vi "Write Focus.vi"(8 "error in (no error)":errorcluster, 10 "GSdevice.lvclass":refnum<class "GSdevice.lvclass">, 11 "GSserver in":refnum<class "GSserver.lvclass">) -> (0 "error out":errorcluster, 3 "GSserver out":refnum<class "GSserver.lvclass">)   [LabVIEW 2018, in "GSserver.lvclass"]
uses:
  GSserver.lvclass
  GSdevice/GSdevice.lvclass
  GSserver.lvclass/GSserver.ctl
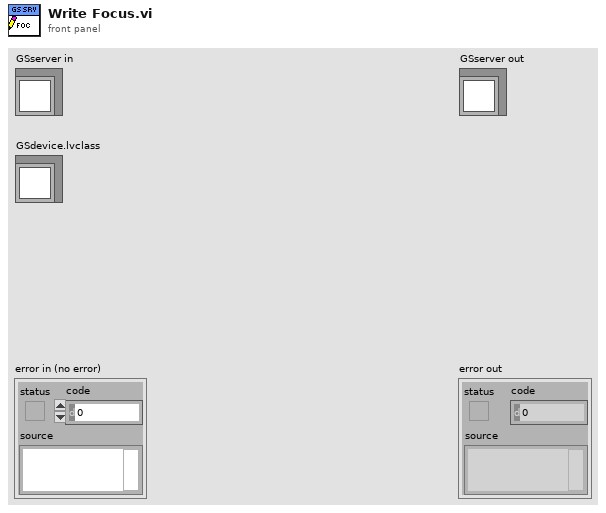
[diagram p1: front panel]
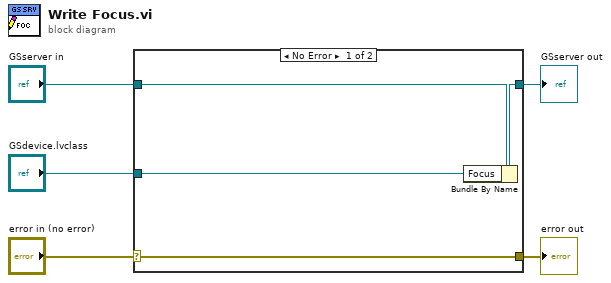
[diagram p0: block diagram]
diagram:
  n1 = case shown="No Error" "error in (no error)" {
    selector: "error in (no error)" -> [w9 w10]
    tunnel: [w9 w10] -> w4
    tunnel: [w7 w11] -> w2
    tunnel: "GSserver in" -> [w8 w11]
    tunnel: "GSdevice.lvclass" -> [w6 _]
    frame No Error {
      n2 = Bundle By Name(cluster=w8, "Focus"=w6) -> (w7:refnum<class "GSserver.lvclass">)
    }
    frame Error {
    }
  }
  "error out" <- w4
  "GSserver out" <- w2
